vi "Select objects in a 3D picture control.vi"() -> ()   [LabVIEW 2010]
uses:
  <vilib>/Utility/miscctls.llb/LV3DPointTypeDef.ctl
  <vilib>/picture/3D Picture Control/NI_3D Picture Control.lvlib
panel:
  out "PickPoint":T1
  out "Selected Object":string
  in  "stop":bool
  out "3D Picture Control":refnum<vi>(3d-picture)
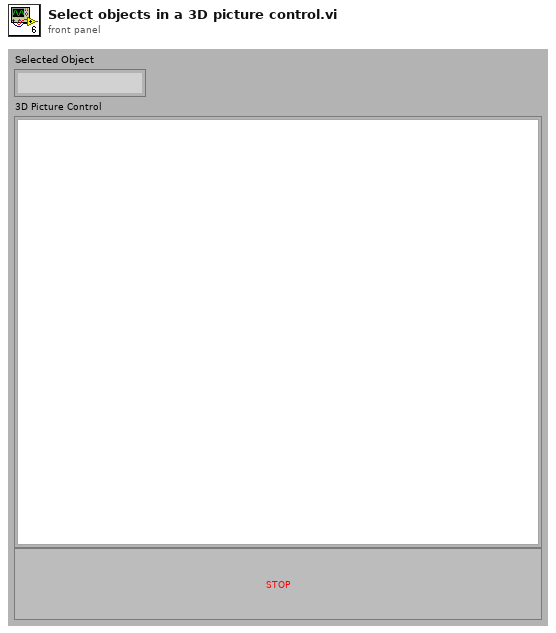
[diagram p1: front panel]
types:
  T1 = typedef "LV3DPointTypeDef.ctl" = cluster{"X":sgl, "Y":sgl, "Z":sgl}
  T2 = cluster{"Red":sgl, "Green":sgl, "Blue":sgl, "Alpha":sgl}
  T3 = typedef "LVPoint32TypeDef.ctl" = cluster{"Horizontal":i32, "Vertical":i32}
  T4 = typedef "LVPositionTypeDef.ctl" = cluster{"Left":i32, "Top":i32}
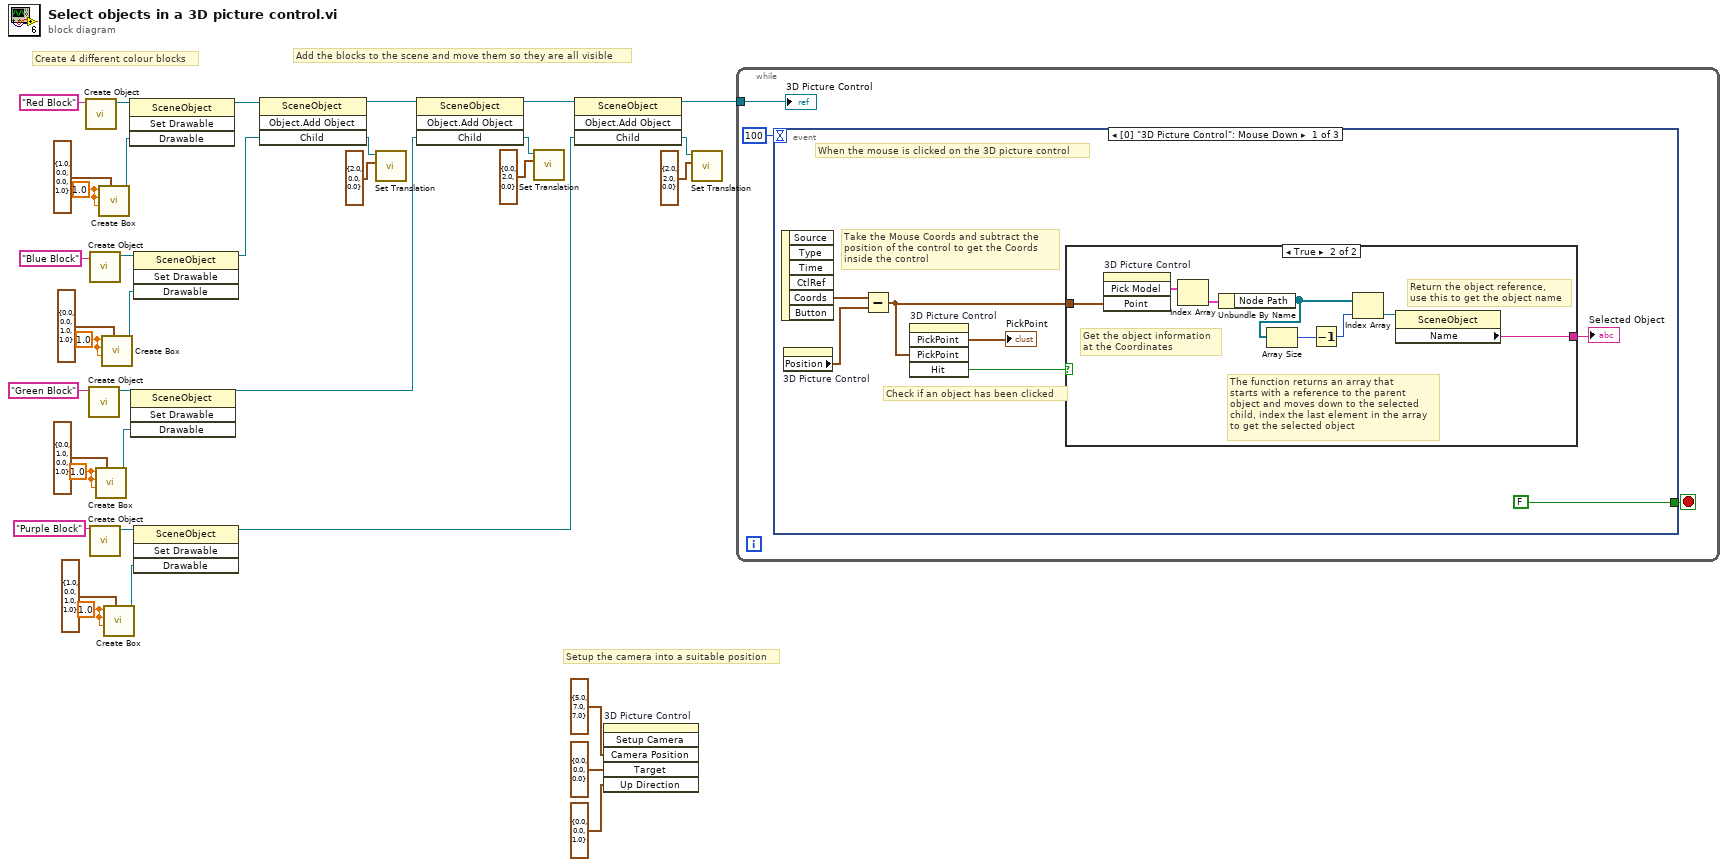
[diagram p0: block diagram]
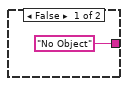
[diagram p2: hidden frame]
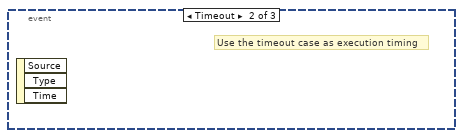
[diagram p3: hidden frame]
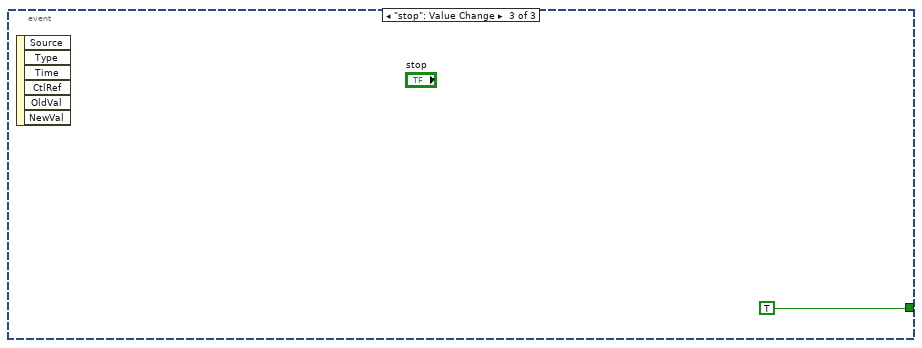
[diagram p4: hidden frame]
diagram:
  w20 = sgl 1.0 ("Length X")
  w27 = sgl 1.0 ("Length X")
  w28 = sgl 1.0 ("Length X")
  w35 = sgl 1.0 ("Length X")
  # "Setup the camera into a suitable position"
  # "Add the blocks to the scene and move them so they are all visible"
  # "Create 4 different colour blocks"
  n1 = call <vilib>:"Create Object.vi"("Name"="Red Block") -> ("Scene:New Object"=w33:refnum<vi>)  [unwired: 1 in, 9 out]
  n2 = call <vilib>:"Create Object.vi"("Name"="Green Block") -> ("Scene:New Object"=w25:refnum<vi>)  [unwired: 1 in, 9 out]
  n3 = call <vilib>:"Create Object.vi"("Name"="Blue Block") -> ("Scene:New Object"=w30:refnum<vi>)  [unwired: 1 in, 9 out]
  n4 = call <vilib>:"Create Object.vi"("Name"="Purple Block") -> ("Scene:New Object"=w22:refnum<vi>)  [unwired: 1 in, 9 out]
  n5 = call <vilib>:"Create Box.vi"("Color"=T2 {"Red"=0.0, "Green"=1.0, "Blue"=0.0, "Alpha"=1.0}, "Length Z"=w27, "Length Y"=w27, "Length X"=w27) -> ("New Box Refnum"=w24:refnum<vi>)  [unwired: 1 in, 6 out]
  n6 = call <vilib>:"Create Box.vi"("Color"=T2 {"Red"=1.0, "Green"=0.0, "Blue"=0.0, "Alpha"=1.0}, "Length Z"=w35, "Length Y"=w35, "Length X"=w35) -> ("New Box Refnum"=w32:refnum<vi>)  [unwired: 1 in, 6 out]
  n7 = call <vilib>:"Create Box.vi"("Color"=T2 {"Red"=0.0, "Green"=0.0, "Blue"=1.0, "Alpha"=1.0}, "Length Z"=w28, "Length Y"=w28, "Length X"=w28) -> ("New Box Refnum"=w31:refnum<vi>)  [unwired: 1 in, 6 out]
  n8 = call <vilib>:"Create Box.vi"("Color"=T2 {"Red"=1.0, "Green"=0.0, "Blue"=1.0, "Alpha"=1.0}, "Length Z"=w20, "Length Y"=w20, "Length X"=w20) -> ("New Box Refnum"=w23:refnum<vi>)  [unwired: 1 in, 6 out]
  n9 = invoke class="SceneObject" method="Set Drawable"(reference=w33, "Drawable"=w32) -> (reference out=w16:refnum<vi>)  [unwired: 2 in, 3 out]
  n10 = invoke class="SceneObject" method="Set Drawable"(reference=w25, "Drawable"=w24) -> (reference out=w1:refnum<vi>)  [unwired: 2 in, 3 out]
  n11 = invoke class="SceneObject" method="Set Drawable"(reference=w30, "Drawable"=w31) -> (reference out=w13:refnum<vi>)  [unwired: 2 in, 3 out]
  n12 = invoke class="SceneObject" method="Set Drawable"(reference=w22, "Drawable"=w23) -> (reference out=w12:refnum<vi>)  [unwired: 2 in, 3 out]
  n13 = invoke class="SceneObject" method="Object.Add Object"(reference=w16, "Child"=w13) -> (reference out=w15:refnum<vi>, "Child"=w11:refnum<vi>)  [unwired: 2 in, 2 out]
  n14 = call <vilib>:"Set Translation.vi"("Translation"=cluster{"X":sgl, "Y":sgl, "Z":sgl} {"X"=2.0, "Y"=0.0, "Z"=0.0}, "Scene Object"=w11) -> ()  [unwired: 1 in, 9 out]
  n15 = invoke class="SceneObject" method="Object.Add Object"(reference=w15, "Child"=w1) -> (reference out=w14:refnum<vi>, "Child"=w10:refnum<vi>)  [unwired: 2 in, 2 out]
  n16 = call <vilib>:"Set Translation.vi"("Translation"=cluster{"X":sgl, "Y":sgl, "Z":sgl} {"X"=0.0, "Y"=2.0, "Z"=0.0}, "Scene Object"=w10) -> ()  [unwired: 1 in, 9 out]
  n17 = invoke class="SceneObject" method="Object.Add Object"(reference=w14, "Child"=w12) -> (reference out=w5:refnum<vi>, "Child"=w9:refnum<vi>)  [unwired: 2 in, 2 out]
  n18 = invoke on="3D Picture Control" class="SceneGraphDisp (strict)" method="Setup Camera"("Camera Position"=T1 {"X"=5.0, "Y"=7.0, "Z"=7.0}, "Target"=T1 {"X"=0.0, "Y"=0.0, "Z"=0.0}, "Up Direction"=T1 {"X"=0.0, "Y"=0.0, "Z"=1.0}) -> ()  [unwired: 3 in, 6 out]
  n19 = call <vilib>:"Set Translation.vi"("Translation"=cluster{"X":sgl, "Y":sgl, "Z":sgl} {"X"=2.0, "Y"=2.0, "Z"=0.0}, "Scene Object"=w9) -> ()  [unwired: 1 in, 9 out]
  n20 = while {
    tunnel: w5 -> [w38]
    stop <- w39 stop-if-true
    n21 = event shown="[0] \"3D Picture Control\": Mouse Down" {
      selector: _ -> [_ _ _]
      dyn-events: _ -> [_ _ _]
      timeout: 100 -> [_ _ _]
      tunnel: [FALSE _ TRUE] -> w39
      event "3D Picture Control": Mouse Down {
        # "Check if an object has been clicked"
        # "Take the Mouse Coords and subtract the\nposition of the control to get the Coords \ninside the control"
        # "When the mouse is clicked on the 3D picture control"
        n22 = event-data() -> ("Coords"=w45:T3)  [unwired: 6 out]
        n23 = property on="3D Picture Control" class="SceneGraphDisp (strict)"() -> ("Position"=w46:T4)  [unwired: 2 in, 2 out]
        n24 = Subtract(x=w45, y=w46) -> (x-y=w42:T3)
        n25 = invoke on="3D Picture Control" class="SceneGraphDisp (strict)" method="PickPoint"("PickPoint"=w42) -> ("PickPoint"=→"PickPoint":T1, "Hit"=w41:bool)  [unwired: 4 in, 3 out]
        n26 = case shown="True" w41 {
          tunnel: w42 -> [_ w55]
          tunnel: ["No Object" ("Name") w48] -> w40
          frame False {
          }
          frame True {
            # "Return the object reference,\nuse this to get the object name"
            # "The function returns an array that\nstarts with a reference to the parent\nobject and moves down to the selected\nchild, index the last element in the array \nto get the selected object"
            # "Get the object information\nat the Coordinates"
            n27 = invoke on="3D Picture Control" class="SceneGraphDisp (strict)" method="Pick Model"("Point"=w55) -> ("Pick Model"=w53:cluster{"Node Path":refnum<vi>[]}[])  [unwired: 3 in, 3 out]
            n28 = Index Array(array=w53) -> (element=w54:cluster{"Node Path":refnum<vi>[]})  [unwired: 1 in]
            n29 = Unbundle By Name(w54) -> ("Node Path"=w52:refnum<vi>[])
            n30 = Array Size(array=w52) -> (size(s)=w50:i32)
            n31 = Decrement(x=w50) -> (x-1=w49:i32)
            n32 = Index Array(array=w52, index=w49) -> (element=w51:refnum<vi>)
            n33 = property class="SceneObject"(reference=w51) -> ("Name"=w48:string)  [unwired: 1 in, 2 out]
          }
        }
        "Selected Object" <- w40
      }
      event Timeout {
        # "Use the timeout case as execution timing"
        n34 = event-data() -> ()  [unwired: 4 out]
      }
      event "stop": Value Change {
        n35 = event-data() -> ()  [unwired: 7 out]
      }
    }
    "3D Picture Control" <- w38
  }
